vi "sub_nextGuess.vi"(9 "invalid guesses":T1[](array[typedef]), 10 "current guess queue":T1[](array[typedef]), 11 "solver array":cluster{"solved":bool, "values":string[]}[][](array[cluster])) -> (1 "no valid guess ?":bool, 2 "next guess":T1, 3 "potential guesses":T1[](array[typedef]))   [LabVIEW 2018]
uses:
  guess.ctl
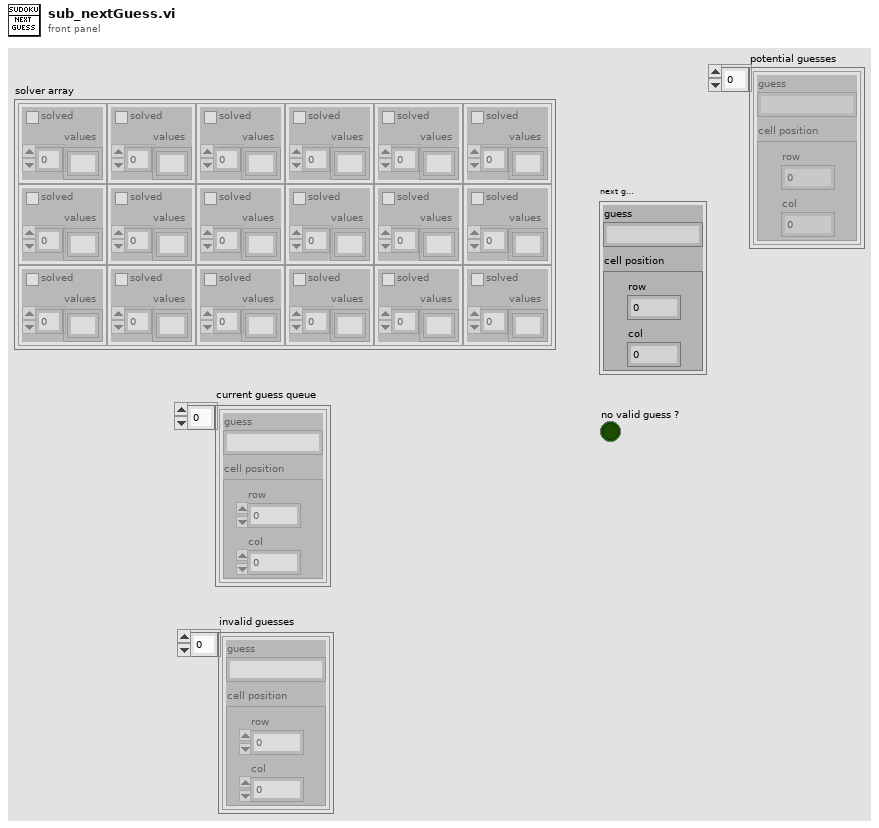
[diagram p1: front panel]
types:
  T1 = typedef "guess.ctl" = cluster{"cell position":cluster{"row":i32, "col":i32}, "guess":string}
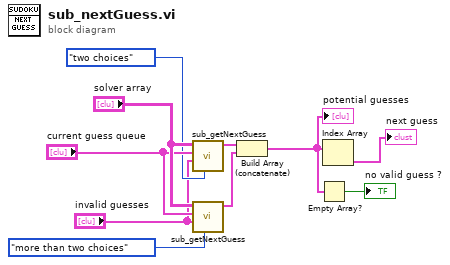
[diagram p0: block diagram]
diagram:
  n1 = call "sub_getNextGuess.vi"("guess candidates"=enum16{"two choices", "more than two choices"}."two choices", "invalid guesses"="invalid guesses", "current guess queue"="current guess queue", "solver array"="solver array") -> ("potential guesses"=w4:T1[])  [unwired: 7 in]
  n2 = call "sub_getNextGuess.vi"("guess candidates"=enum16{"two choices", "more than two choices"}."more than two choices", "invalid guesses"="invalid guesses", "current guess queue"="current guess queue", "solver array"="solver array") -> ("potential guesses"=w3:T1[])  [unwired: 7 in]
  n3 = Build Array (concatenate)(w4, w3) -> (w1:T1[])
  "potential guesses" <- w1
  n4 = Empty Array?(array=w1) -> (empty?=→"no valid guess ?":bool)
  n5 = Index Array(array=w1) -> (element=→"next guess":T1)  [unwired: 1 in]
